vi "公式.vi"(7 "功能":enum16{"读取", "写入"}(ring), 8 "error in (no error)":errorcluster caption="错误输入（无错误）", 10 "公式写入":cluster{"X^2":dbl, "X":dbl, "b":dbl}, 11 "MB session in":refnum<class "MB_Master.lvclass">) -> (0 "error out":errorcluster caption="错误输出", 2 "公式读取":cluster{"X^2":dbl, "X":dbl, "b":dbl}, 3 "MB session out":refnum<class "MB_Master.lvclass">)   [LabVIEW 2016, in "斯坦道氟化物.lvlib"]
uses:
  <vilib>/Plasmionique/MB Master/MB_Master/MB_Master.lvclass
  <vilib>/Plasmionique/MB Master/MB Master.lvlib
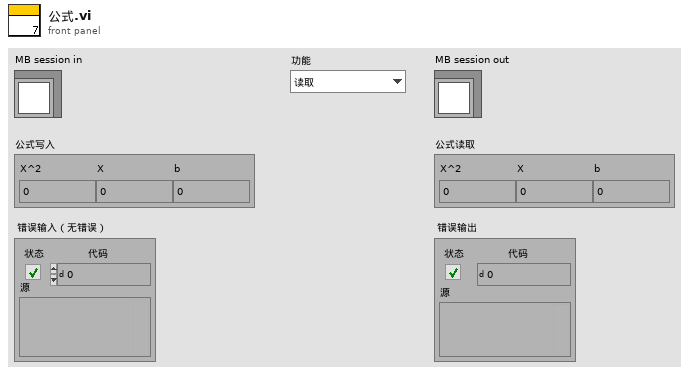
[diagram p1: front panel]
types:
  T1 = typedef "SingleStepTestV3.lvlib/SingleStepTestV3.lvclass/仪器版本.ctl" = enum16{"V3.1版", "V4版", "V3版", "V4.2版"}
  T2 = cluster{"FLOAT[0]":sgl, "FLOAT[1]":sgl, "FLOAT[2]":sgl}
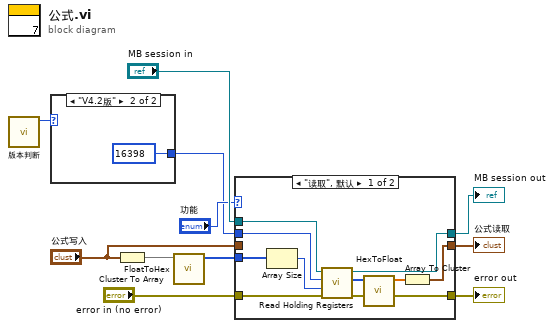
[diagram p0: block diagram]
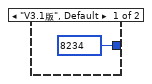
[diagram p2: hidden frame]
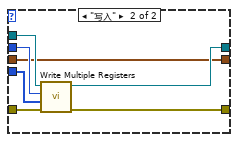
[diagram p3: hidden frame]
diagram:
  n1 = call "版本判断.vi"() -> ("仪器版本"=w3:T1)  [unwired: 11 in]
  n2 = case shown="\"V4.2版\"" w3 {
    tunnel: [u16 8234 ("starting address") u16 16398 ("starting address")] -> w2
    frame "V3.1版", Default {
    }
    frame "V4.2版" {
    }
  }
  n3 = Cluster To Array(cluster="公式写入") -> (array=w9:dbl[])
  n4 = call "FloatToHex.vi"("浮点数"=w9) -> ("DCBA整形输出"=w8:u16[])  [unwired: 10 in]
  n5 = case shown="\"读取\", 默认" "功能" {
    tunnel: "error in (no error)" -> [w20 w30]
    tunnel: [w21 w29] -> w10
    tunnel: [w22 w28] -> w1
    tunnel: w2 -> [w19 w27]
    tunnel: w8 -> [w18 w26]
    tunnel: "MB session in" -> [w23 w25]
    tunnel: [w14 w24] -> w4
    tunnel: "公式写入" -> [_ w24]
    frame "读取", Default {
      n6 = Array Size(array=w18) -> (size(s)=w17:i32)
      n7 = call <vilib>:"Read Holding Registers.vi"("error in (no error)"=w20, "quantity"=w17, "starting address"=w19, "MB session in"=w23) -> ("error out"=w21:errorcluster, "Registers"=w15:u16[], "MB session out"=w22:refnum<class "MB_Master.lvclass">)  [unwired: 5 in]
      n8 = call "HexToFloat.vi"("数组"=w15) -> ("FLOAT"=w16:sgl[])  [unwired: 10 in]
      n9 = Array To Cluster(array=w16) -> (cluster=w14:T2)
    }
    frame "写入" {
      n10 = call <vilib>:"Write Multiple Registers.vi"("error in (no error)"=w30, "values"=w26, "starting address"=w27, "MB session in"=w25) -> ("error out"=w29:errorcluster, "MB session out"=w28:refnum<class "MB_Master.lvclass">)  [unwired: 6 in]
    }
  }
  "error out" <- w10
  "MB session out" <- w1
  "公式读取" <- w4
